vi "http vi.vi"() -> ()   [LabVIEW 2011]
panel:
  out "HTTP Length":i32
  in  "循环计数值":i32
  in  "HTTP Body":string
  in  "HTTP Header":string
  out "HTTP File":string
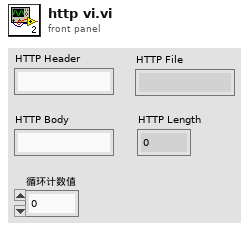
[diagram p1: front panel]
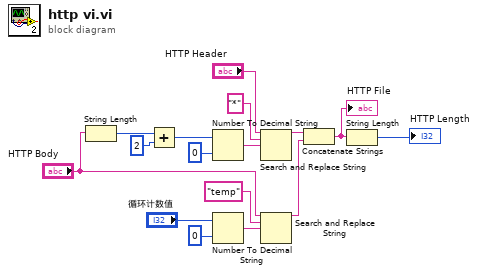
[diagram p0: block diagram]
diagram:
  n1 = String Length ("字符串长度")(string="HTTP Body") -> (length=w9:i32)
  n2 = Add(x=w9, y=2 ("计数值增量")) -> (x+y=w12:i32)
  n3 = Number To Decimal String(number=w12, width (-)=u16 0 ("宽度(-)")) -> (decimal integer string=w13:string)
  n4 = Number To Decimal String(number="循环计数值", width (-)=u16 0 ("宽度(-)")) -> (decimal integer string=w5:string)
  n5 = Search and Replace String ("搜索替换字符串")(input string="HTTP Header", search string="*" ("搜索字符串"), replace string=w13) -> (result string=w14:string)  [unwired: 5 in, 3 out]
  n6 = Search and Replace String(input string="HTTP Body", search string="temp" ("搜索字符串"), replace string=w5) -> (result string=w15:string)  [unwired: 5 in, 3 out]
  n7 = Concatenate Strings(w14, w15) -> (w16:string)
  "HTTP File" <- w16
  n8 = String Length(string=w16) -> (length=→"HTTP Length":i32)
